vi "Simulate Mechanical Action.vi"(4 "Error In":errorcluster, 7 "Button CtlRef":refnum<vi>) -> (0 "Error Out":errorcluster)   [LabVIEW 2014, in "User Interface.lvlib"]
uses:
  User Interface.lvlib
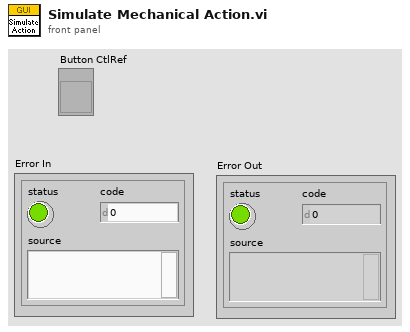
[diagram p1: front panel]
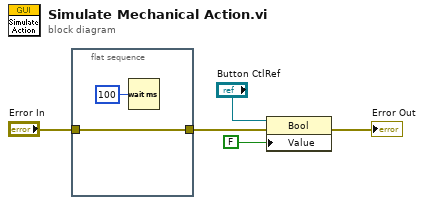
[diagram p0: block diagram]
diagram:
  n1 = flat-sequence {
    tunnel: "Error In" -> [w6]
    tunnel: [w6] -> w4
    frame #0 {
      n2 = Wait (ms)(milliseconds to wait=u32 100) -> ()  [unwired: 1 out]
    }
  }
  n3 = property class="Bool"(reference="Button CtlRef", error in=w4, "Value"=FALSE) -> (error out=→"Error Out":errorcluster)  [unwired: 1 out]
